vi "Add Probes to all wires.vi"(8 "error in":errorcluster, 11 "VI Refnum In":refnum<vi>) -> (0 "error out":errorcluster, 3 "VI Refnum Out":refnum<vi>)   [LabVIEW 2020]
doc: "Add probes to all wires of the active VI."
uses:
  <vilib>/Utility/traverseref.llb/TRef TravTarget.ctl
  src/Type Definitions/Class Name--enum.ctl
  <vilib>/Utility/traverseref.llb/VI Scripting - Traverse.lvlib
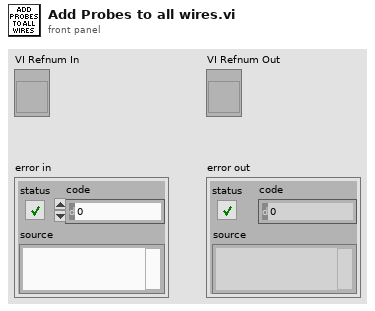
[diagram p1: front panel]
types:
  T1 = typedef "Class Name--enum.ctl" = enum16{"Node", "Wire"}
  T2 = typedef "TRef TravTarget.ctl" = enum16{"FP", "BD", "Other"}
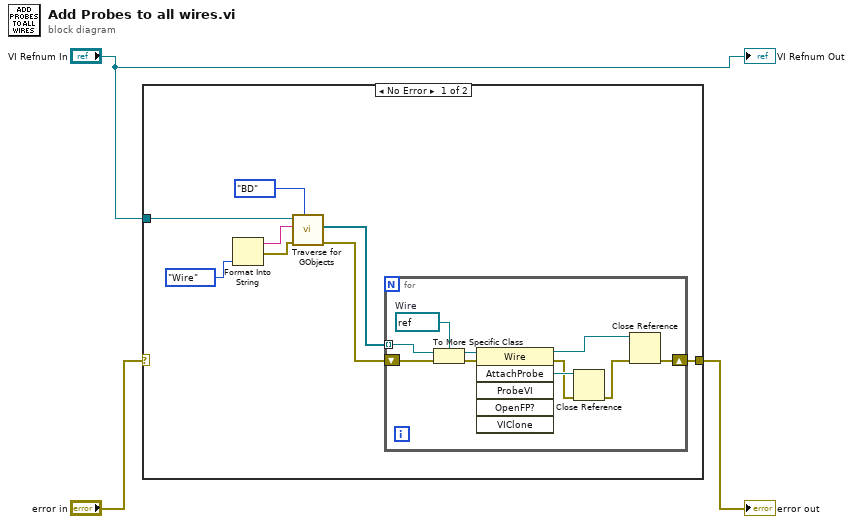
[diagram p0: block diagram]
diagram:
  n1 = case shown="No Error" "error in" {
    selector: "error in" -> [_ w22]
    tunnel: [w11 w22] -> w2
    tunnel: "VI Refnum In" -> [w4 _]
    frame No Error {
      n2 = Format Into String(Class_Name--enum."Wire" ("input 1")) -> (resulting string=w8:string, error out=w10:errorcluster)  [unwired: 3 in]
      n3 = call <vilib>:"Traverse for GObjects.vi"("Traverse Target"=TRef_TravTarget."BD", "error in (no error)"=w10, "Class Name"=w8, "VI Refnum"=w4) -> ("error out"=w9:errorcluster, "References"=w5:refnum<vi>[])  [unwired: 4 in, 2 out]
      n4 = for {
        tunnel: w5 -> [w18] mode=indexing
        shift-right: [w19] -> w11
        shift-left: w9 -> [w21]
        w16 = refnum<vi> refnum  # Wire
        n5 = To More Specific Class(target class=w16, reference=w18, error in=w21) -> (specific class reference=w17:refnum<vi>, error out=w20:errorcluster)
        n6 = invoke class="Wire" method="AttachProbe"(reference=w17, error in=w20) -> (reference out=w15:refnum<vi>, error out=w13:errorcluster, "Attach Probe"=w14:refnum<vi>)  [unwired: 4 in, 3 out]
        n7 = Close Reference(reference=w14, error in (no error)=w13) -> (error out=w12:errorcluster)
        n8 = Close Reference(reference=w15, error in (no error)=w12) -> (error out=w19:errorcluster)
      }
    }
    frame Error {
      # "Pass error without further action"
    }
  }
  "error out" <- w2
  "VI Refnum Out" <- "VI Refnum In"
